vi "Read Last Waveform.vi"(8 "error in (no error)":errorcluster, 10 "Channel":u8, 11 "Scope Base in":refnum<class "Scope Base.lvclass">) -> (0 "error out":errorcluster, 2 "Last Waveform":waveform(dbl), 3 "Scope Base out":refnum<class "Scope Base.lvclass">)   [LabVIEW 2023, in "HAL.lvlib" / "Scope Base.lvlib" / "Scope Base.lvclass"]
uses:
  Scope Base.lvclass
  Scope Base.lvclass/Scope Base.ctl
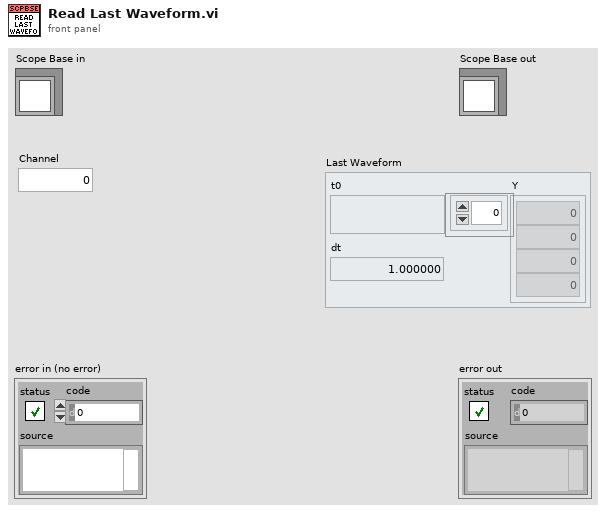
[diagram p1: front panel]
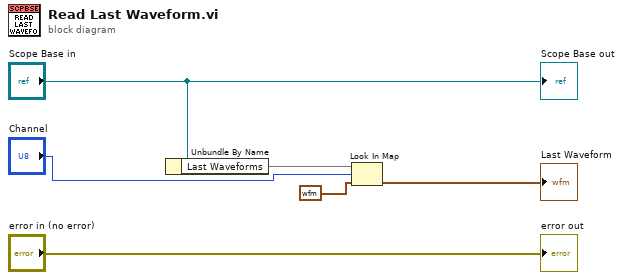
[diagram p0: block diagram]
diagram:
  n1 = Unbundle By Name("Scope Base in") -> ("Last Waveforms"=w4:map{u8, waveform(dbl)})
  n2 = Look In Map(map=w4, key="Channel", default value=waveform(dbl) {"t0"=timestamp(0 s since 1904-01-01), "dt"=1.0, "Y"=[]} ("Waveform")) -> (value=→"Last Waveform":waveform(dbl))  [unwired: 1 out]
  "error out" <- "error in (no error)"
  "Scope Base out" <- "Scope Base in"
